vi "QuantumX_Device.vi"(4 "StreamingPort":i32=7411, 5 "HttpPort":i32=80, 6 "Error in":errorcluster, 7 "Port":i32=5001, 8 "IPAddress":string) -> (0 "Error out":errorcluster, 3 "Device":refnum<k24>)   [LabVIEW 2016]
doc: "Generates a new QuantumX device.\n\nIPAddress: IPAddress of the device you want to connect with\nPort: Port of the device you want to connect with (default port is 5001)\nHttpPort: Http port of the device (default is 80)\nStreamingPort: Port that is used for streaming (default is 7411)"
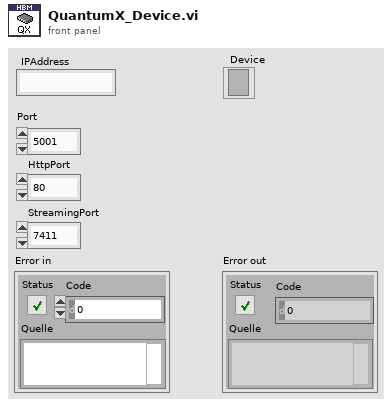
[diagram p1: front panel]
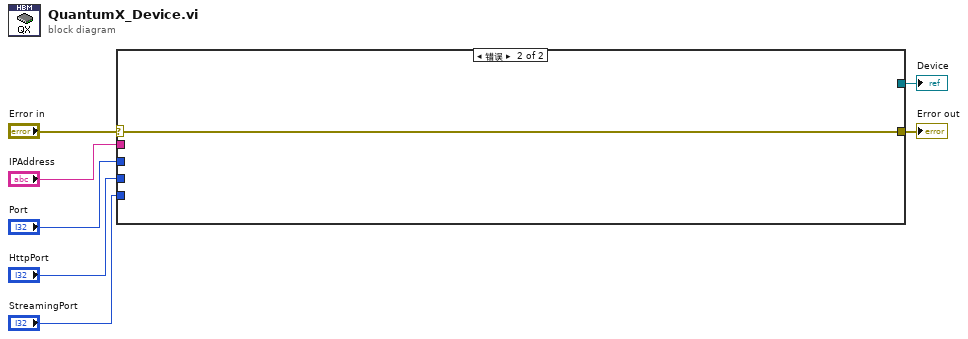
[diagram p0: block diagram]
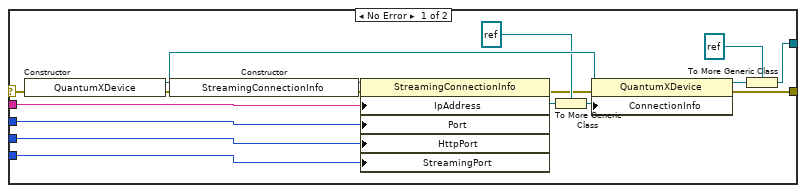
[diagram p2: hidden frame]
diagram:
  n1 = case shown="错误" "Error in" {
    selector: "Error in" -> [w19 w25]
    tunnel: "IPAddress" -> [w17 _]
    tunnel: "Port" -> [w16 _]
    tunnel: [w9 w25] -> w4
    tunnel: [w20 _] -> w3
    tunnel: "StreamingPort" -> [w15 _]
    tunnel: "HttpPort" -> [w14 _]
    frame No Error {
      n2 = constructor class="QuantumXDevice"(error in=w19) -> (reference out=w23:refnum<k24>, error out=w24:errorcluster)  [unwired: 2 in, 1 out]
      n3 = constructor class="StreamingConnectionInfo"(error in=w24) -> (reference out=w18:refnum<k24>, error out=w13:errorcluster)  [unwired: 2 in, 1 out]
      n4 = property on="Eigenschaftsknoten" class="StreamingConnectionInfo"(reference=w18, error in=w13, "IpAddress"=w17, "Port"=w16, "HttpPort"=w14, "StreamingPort"=w15) -> (reference out=w12:refnum<k24>, error out=w10:errorcluster)
      n5 = To More Generic Class(target class=refnum<k24> refnum (".NET (Referenz)"), reference=w12) -> (generic class reference=w22:refnum<k24>)
      n6 = property on="Eigenschaftsknoten" class="QuantumXDevice"(reference=w23, error in=w10, "ConnectionInfo"=w22) -> (reference out=w21:refnum<k24>, error out=w9:errorcluster)
      n7 = To More Generic Class(target class=refnum<k24> refnum (".NET (Referenz)"), reference=w21) -> (generic class reference=w20:refnum<k24>)
    }
    frame Error {
    }
  }
  "Error out" <- w4
  "Device" <- w3
